vi "7SegmentProgramMarcoGonzalez.vi"() -> ()   [LabVIEW 2012]
panel:
  out "8":bool
  out "7":bool
  out "6":bool
  out "5":bool
  out "4":bool
  out "3":bool
  out "2":bool
  out "1":bool
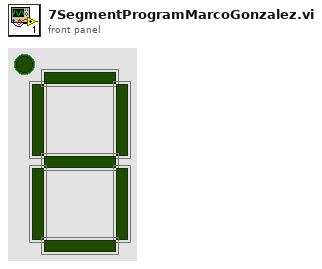
[diagram p1: front panel]
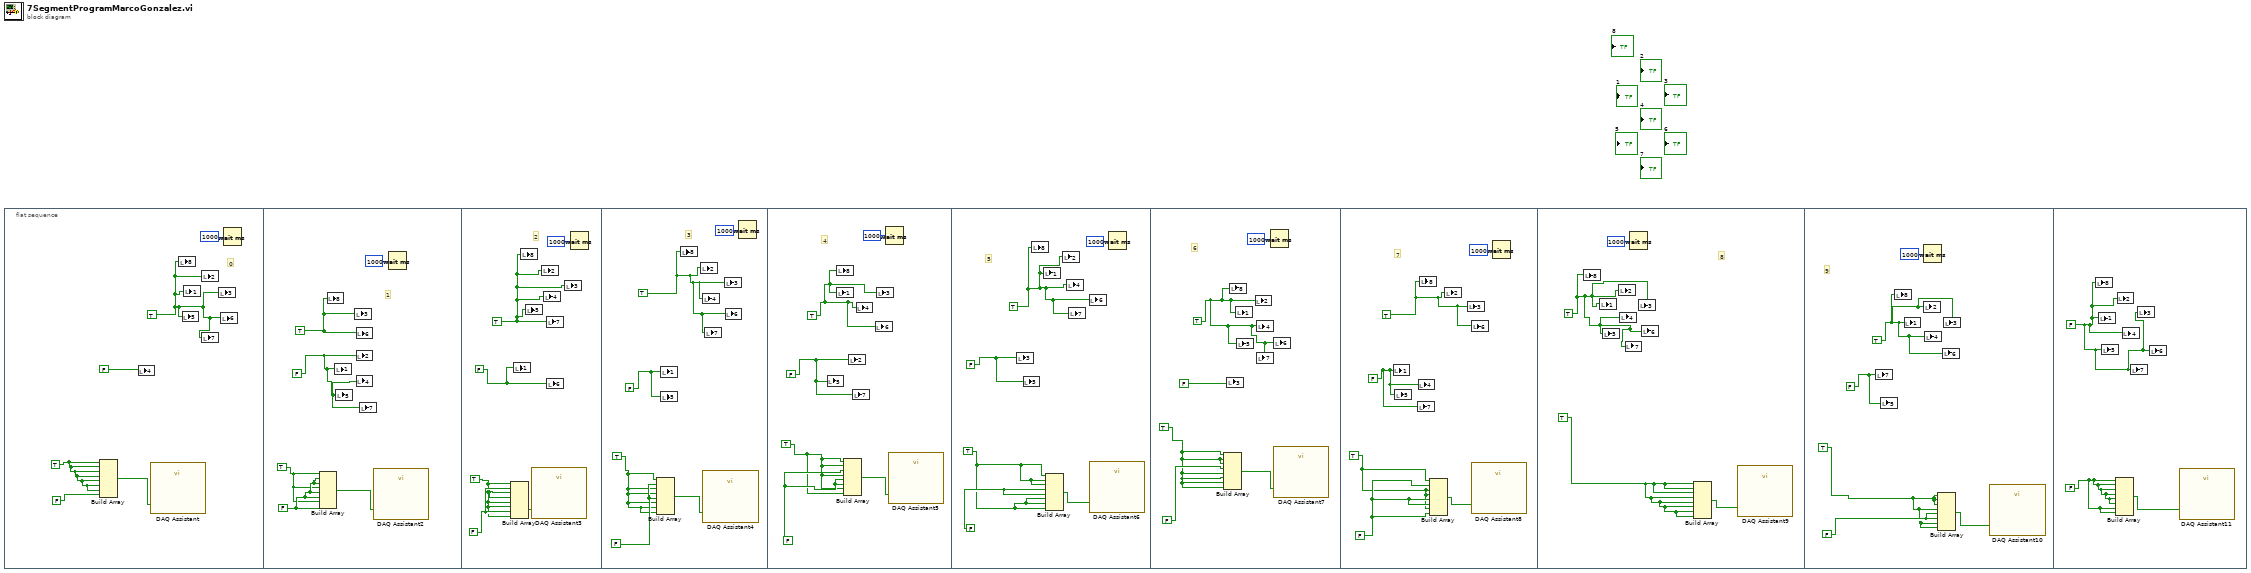
[diagram p0: block diagram]
diagram:
  n1 = flat-sequence {
    frame #0 {
      w2 = TRUE
      w6 = TRUE
      # "0"
      n2 = Build Array(w2, w2, w2, w2, w2, w2, w2, FALSE) -> (w1:bool[])
      n3 = local write "4"(FALSE) -> ()
      n4 = call "DAQ Assistant"("data"=w1) -> ()  [unwired: 17 in, 2 out]
      n5 = local write "8"(w6) -> ()
      n6 = local write "5"(w6) -> ()
      n7 = local write "1"(w6) -> ()
      n8 = local write "2"(w6) -> ()
      n9 = local write "7"(w6) -> ()
      n10 = local write "3"(w6) -> ()
      n11 = local write "6"(w6) -> ()
      n12 = Wait (ms)(milliseconds to wait=u32 1000) -> ()  [unwired: 1 out]
    }
    frame #1 {
      w9 = FALSE
      w7 = TRUE
      w10 = FALSE
      w12 = TRUE
      # "1"
      n13 = Build Array(w7, w9, w9, w7, w9, w9, w7, w9) -> (w8:bool[])
      n14 = local write "8"(w12) -> ()
      n15 = local write "1"(w10) -> ()
      n16 = local write "5"(w10) -> ()
      n17 = local write "3"(w12) -> ()
      n18 = local write "6"(w12) -> ()
      n19 = local write "2"(w10) -> ()
      n20 = local write "4"(w10) -> ()
      n21 = local write "7"(w10) -> ()
      n22 = call "DAQ Assistant2"("data"=w8) -> ()  [unwired: 17 in, 2 out]
      n23 = Wait (ms)(milliseconds to wait=u32 1000) -> ()  [unwired: 1 out]
    }
    frame #2 {
      w15 = FALSE
      w13 = TRUE
      w16 = FALSE
      w18 = TRUE
      # "2"
      n24 = Build Array(w13, w15, w13, w13, w13, w13, w15, w13) -> (w14:bool[])
      n25 = local write "1"(w16) -> ()
      n26 = local write "8"(w18) -> ()
      n27 = local write "5"(w18) -> ()
      n28 = call "DAQ Assistant3"("data"=w14) -> ()  [unwired: 17 in, 2 out]
      n29 = local write "2"(w18) -> ()
      n30 = local write "4"(w18) -> ()
      n31 = local write "7"(w18) -> ()
      n32 = local write "6"(w16) -> ()
      n33 = local write "3"(w18) -> ()
      n34 = Wait (ms)(milliseconds to wait=u32 1000) -> ()  [unwired: 1 out]
    }
    frame #3 {
      w21 = FALSE
      w19 = TRUE
      w22 = FALSE
      w24 = TRUE
      # "3"
      n35 = Build Array(w19, w21, w19, w19, w21, w19, w19, w19) -> (w20:bool[])
      n36 = local write "1"(w22) -> ()
      n37 = local write "5"(w22) -> ()
      n38 = local write "8"(w24) -> ()
      n39 = local write "2"(w24) -> ()
      n40 = local write "4"(w24) -> ()
      n41 = call "DAQ Assistant4"("data"=w20) -> ()  [unwired: 17 in, 2 out]
      n42 = local write "7"(w24) -> ()
      n43 = local write "3"(w24) -> ()
      n44 = local write "6"(w24) -> ()
      n45 = Wait (ms)(milliseconds to wait=u32 1000) -> ()  [unwired: 1 out]
    }
    frame #4 {
      w27 = FALSE
      w25 = TRUE
      w28 = FALSE
      w29 = TRUE
      # "4"
      n46 = local write "5"(w28) -> ()
      n47 = local write "1"(w29) -> ()
      n48 = local write "8"(w29) -> ()
      n49 = Build Array(w25, w25, w27, w25, w27, w27, w25, w25) -> (w26:bool[])
      n50 = local write "2"(w28) -> ()
      n51 = local write "7"(w28) -> ()
      n52 = local write "4"(w29) -> ()
      n53 = local write "6"(w29) -> ()
      n54 = local write "3"(w29) -> ()
      n55 = Wait (ms)(milliseconds to wait=u32 1000) -> ()  [unwired: 1 out]
      n56 = call "DAQ Assistant5"("data"=w26) -> ()  [unwired: 17 in, 2 out]
    }
    frame #5 {
      w33 = FALSE
      w32 = TRUE
      w34 = FALSE
      w36 = TRUE
      # "5"
      n57 = local write "3"(w34) -> ()
      n58 = local write "5"(w34) -> ()
      n59 = local write "8"(w36) -> ()
      n60 = local write "1"(w36) -> ()
      n61 = Build Array(w32, w32, w32, w33, w33, w32, w32, w32) -> (w31:bool[])
      n62 = local write "2"(w36) -> ()
      n63 = local write "4"(w36) -> ()
      n64 = local write "7"(w36) -> ()
      n65 = local write "6"(w36) -> ()
      n66 = call "DAQ Assistant6"("data"=w31) -> ()  [unwired: 17 in, 2 out]
      n67 = Wait (ms)(milliseconds to wait=u32 1000) -> ()  [unwired: 1 out]
    }
    frame #6 {
      w38 = TRUE
      w41 = TRUE
      # "6"
      n68 = Build Array(w38, w38, w38, FALSE, w38, w38, w38, w38) -> (w37:bool[])
      n69 = local write "3"(FALSE) -> ()
      n70 = local write "8"(w41) -> ()
      n71 = local write "1"(w41) -> ()
      n72 = local write "5"(w41) -> ()
      n73 = local write "2"(w41) -> ()
      n74 = local write "4"(w41) -> ()
      n75 = local write "7"(w41) -> ()
      n76 = Wait (ms)(milliseconds to wait=u32 1000) -> ()  [unwired: 1 out]
      n77 = local write "6"(w41) -> ()
      n78 = call "DAQ Assistant7"("data"=w37) -> ()  [unwired: 17 in, 2 out]
    }
    frame #7 {
      w44 = FALSE
      w43 = TRUE
      w46 = FALSE
      w47 = TRUE
      # "7"
      n79 = local write "1"(w46) -> ()
      n80 = local write "5"(w46) -> ()
      n81 = local write "7"(w46) -> ()
      n82 = local write "4"(w46) -> ()
      n83 = local write "8"(w47) -> ()
      n84 = Build Array(w43, w44, w43, w43, w44, w44, w43, w44) -> (w45:bool[])
      n85 = local write "2"(w47) -> ()
      n86 = local write "3"(w47) -> ()
      n87 = local write "6"(w47) -> ()
      n88 = call "DAQ Assistant8"("data"=w45) -> ()  [unwired: 17 in, 2 out]
      n89 = Wait (ms)(milliseconds to wait=u32 1000) -> ()  [unwired: 1 out]
    }
    frame #8 {
      w50 = TRUE
      w52 = TRUE
      # "8"
      n90 = local write "8"(w52) -> ()
      n91 = local write "1"(w52) -> ()
      n92 = local write "5"(w52) -> ()
      n93 = local write "2"(w52) -> ()
      n94 = local write "4"(w52) -> ()
      n95 = local write "7"(w52) -> ()
      n96 = Wait (ms)(milliseconds to wait=u32 1000) -> ()  [unwired: 1 out]
      n97 = local write "3"(w52) -> ()
      n98 = local write "6"(w52) -> ()
      n99 = Build Array(w50, w50, w50, w50, w50, w50, w50, w50) -> (w49:bool[])
      n100 = call "DAQ Assistant9"("data"=w49) -> ()  [unwired: 17 in, 2 out]
    }
    frame #9 {
      w55 = FALSE
      w54 = TRUE
      w56 = FALSE
      w58 = TRUE
      # "9"
      n101 = local write "7"(w56) -> ()
      n102 = local write "5"(w56) -> ()
      n103 = local write "8"(w58) -> ()
      n104 = local write "1"(w58) -> ()
      n105 = Wait (ms)(milliseconds to wait=u32 1000) -> ()  [unwired: 1 out]
      n106 = local write "2"(w58) -> ()
      n107 = local write "4"(w58) -> ()
      n108 = Build Array(w54, w54, w54, w54, w55, w55, w54, w54) -> (w53:bool[])
      n109 = local write "6"(w58) -> ()
      n110 = local write "3"(w58) -> ()
      n111 = call "DAQ Assistant10"("data"=w53) -> ()  [unwired: 17 in, 2 out]
    }
    frame #10 {
      w60 = FALSE
      w61 = FALSE
      n112 = local write "8"(w61) -> ()
      n113 = local write "1"(w61) -> ()
      n114 = local write "5"(w61) -> ()
      n115 = Build Array(w60, w60, w60, w60, w60, w60, w60, w60) -> (w59:bool[])
      n116 = local write "2"(w61) -> ()
      n117 = local write "4"(w61) -> ()
      n118 = local write "7"(w61) -> ()
      n119 = local write "3"(w61) -> ()
      n120 = local write "6"(w61) -> ()
      n121 = call "DAQ Assistant11"("data"=w59) -> ()  [unwired: 17 in, 2 out]
    }
  }
